vi "Get Device Info.vi"(1 "Read Data":string) -> (0 "Device Info":string)   [LabVIEW 2020]
panel:
  out "array":string[](array[string])
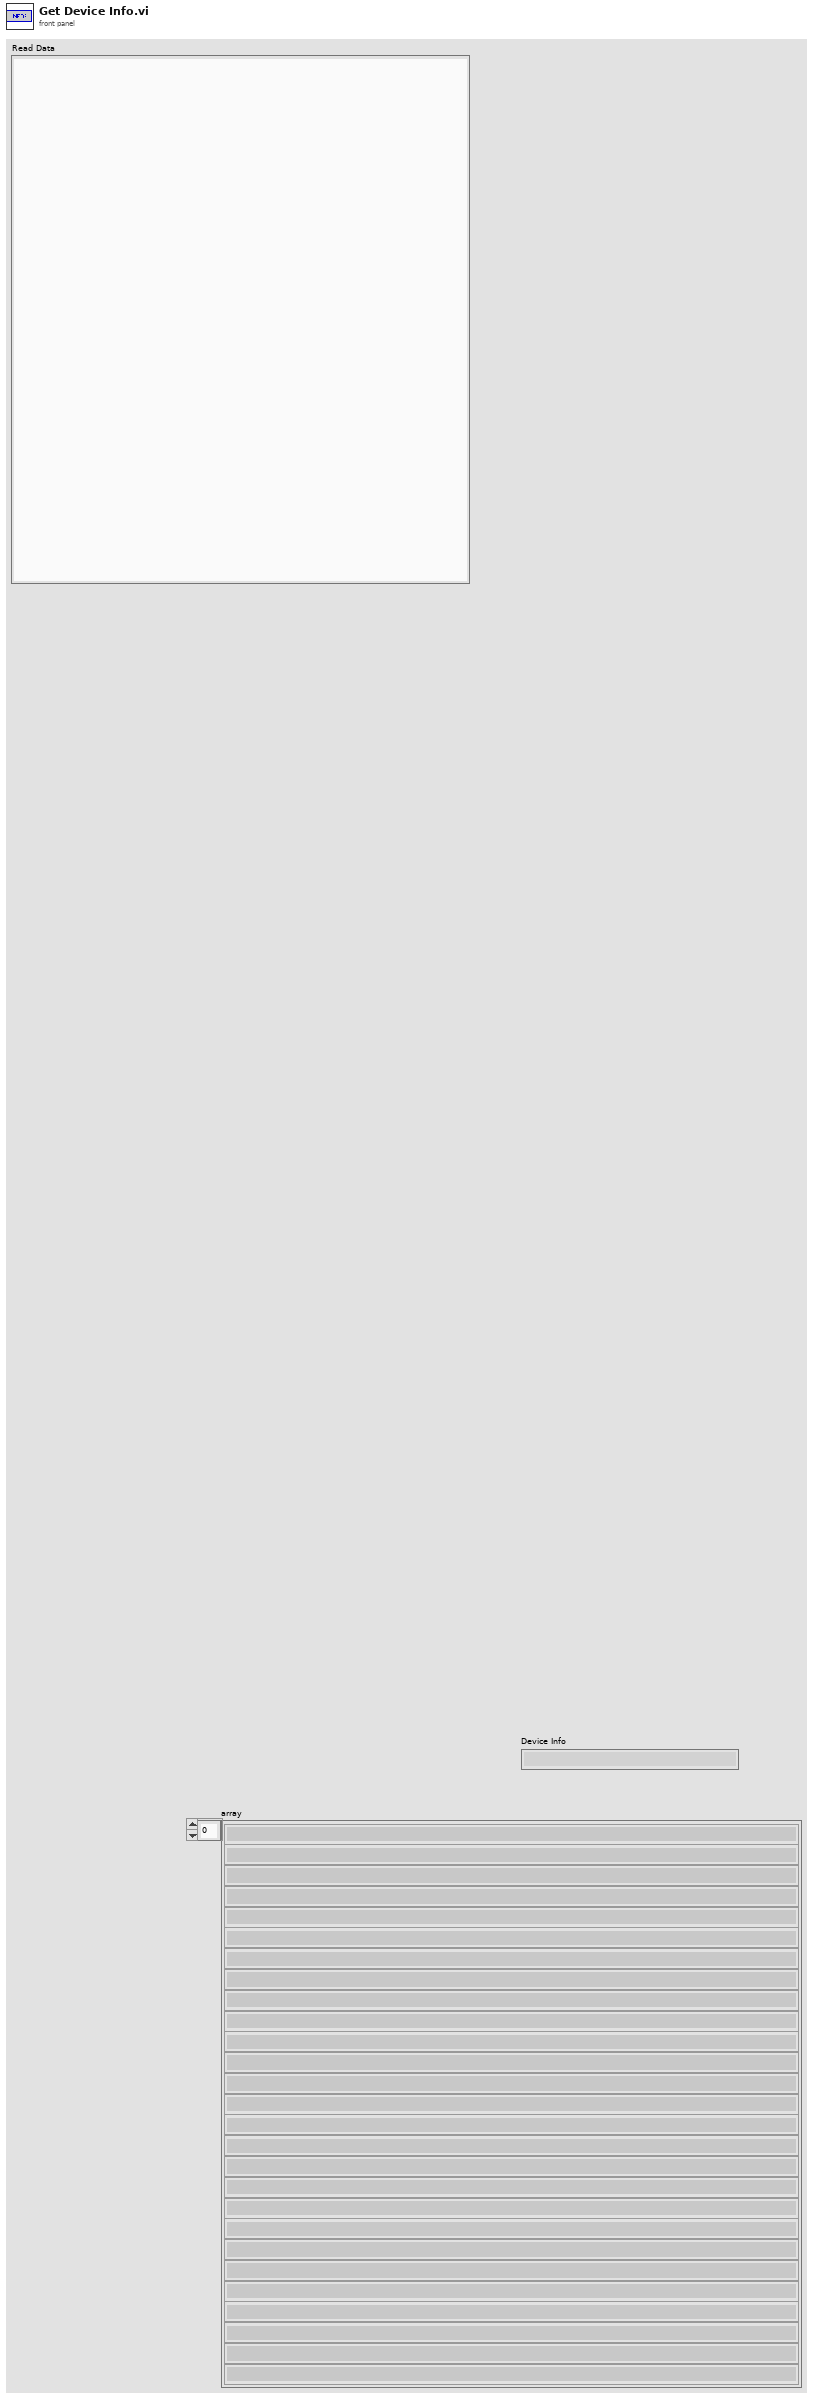
[diagram p1: front panel]
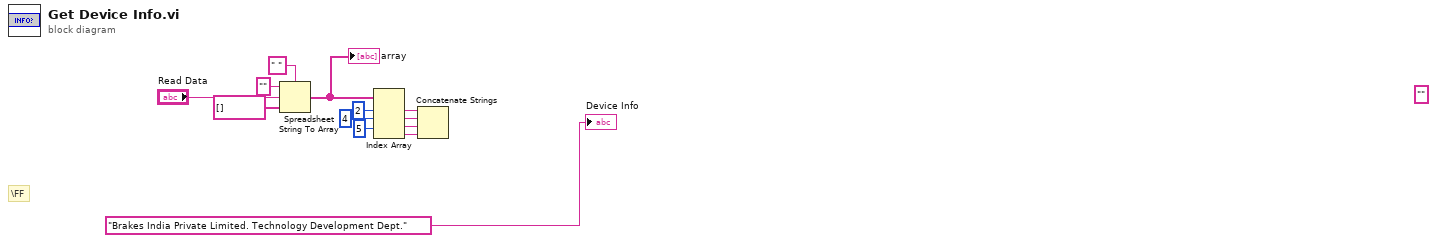
[diagram p0: block diagram]
diagram:
  (unwired) "" ("Read Data")
  # "\\FF"
  n1 = Spreadsheet String To Array(delimiter (Tab)=" ", format string="", spreadsheet string="Read Data", array type (2D Dbl)=string[] []) -> (array=w9:string[])
  "array" <- w9
  n2 = Index Array(array=w9, index #1=2 ("index"), index #2=4 ("index"), index #3=5 ("index")) -> (element #1=w8:string, element #2=w4:string, element #3=w3:string, element #4=w2:string)  [unwired: 1 in]
  n3 = Concatenate Strings(w8, w4, w3, w2) -> ()  [unwired: 1 out]
  "Device Info" <- "Brakes India Private Limited. Technology Development Dept." ("Device Info")
